vi "IMAQSetupBufferList.vi"(10 "IMAQ Session In":refnum<k11>, 11 "Camera":T1={"Framerate (Hz)"=0, "Exposure time (us)"=0, "Image size"={"Width"=1280, "Height"=1024}, "Number of buffers"=30}) -> (3 "IMAQ Refnum out":refnum<k11>)   [LabVIEW 2011]
uses:
  Main/Camera/GenericCameraConfigType.ctl
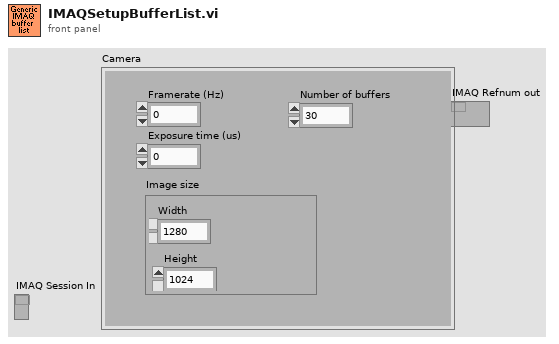
[diagram p1: front panel]
types:
  T1 = typedef "GenericCameraConfigType.ctl" = cluster{"Framerate (Hz)":i32, "Exposure time (us)":i32, "Image size":cluster{"Width":i32, "Height":i32}, "Number of buffers":i32}
  T2 = typedef "Image Type" = u32
  T3 = typedef "IMAQ Image.ctl" = refnum<image>
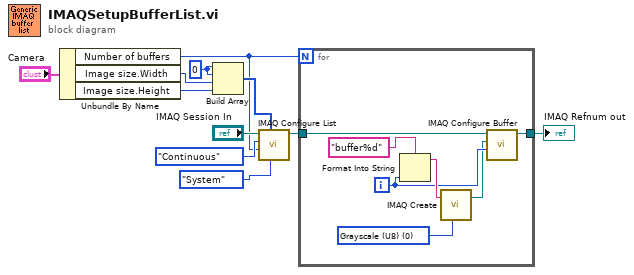
[diagram p0: block diagram]
diagram:
  w5 = 0
  n1 = Unbundle By Name("Camera") -> ("Number of buffers"=w1:i32, "Image size.Width"=w4:i32, "Image size.Height"=w3:i32)
  n2 = Build Array(w5, w5, w4, w3) -> (w6:i32[])
  n3 = call <vilib>:"IMAQ Configure List.vi"("Memory Location"=enum16{"System", "Onboard"}."System", "Region of interest"=w6, "Number of buffers"=w1, "Continuous?"=enum16{"One-Shot", "Continuous"}."Continuous", "IMAQ Session In"="IMAQ Session In") -> ("IMAQ Session Out"=w11:refnum<k11>)  [unwired: 1 in, 5 out]
  n4 = for {
    N: w1 -> [_]
    tunnel: w11 -> [w15]
    tunnel: [w14] -> w8
    i -> [w16]
    w13 = T2 0 items=["Grayscale (U8)", "Grayscale (I16)", "Grayscale (SGL)", "Complex (CSG)", "RGB (U32)", "HSL (U32)", "RGB (U64)", "Grayscale (U16)"] ("Image Type")
    n5 = Format Into String(format string="buffer%d", w16) -> (resulting string=w17:string)  [unwired: 2 in, 1 out]
    n6 = call "IMAQ Create"("Image Name"=w17, "Image Type"=w13) -> ("New Image"=w12:T3)  [unwired: 2 in, 2 out]
    n7 = call <vilib>:"IMAQ Configure Buffer.vi"("Buffer Number"=w16, "Image In"=w12, "IMAQ Session In"=w15) -> ("IMAQ Session Out"=w14:refnum<k11>)  [unwired: 3 in, 5 out]
  }
  "IMAQ Refnum out" <- w8
